vi "BPVI.vi"() -> ()   [LabVIEW 2014]
panel:
  in  "Array":void[](array[numeric])
  in  "Z-Expected":dbl
  in  "Y-Expected":dbl
  in  "X-Expected":dbl
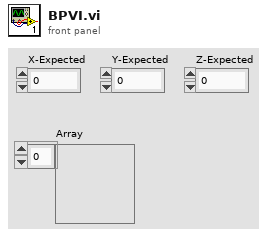
[diagram p1: front panel]
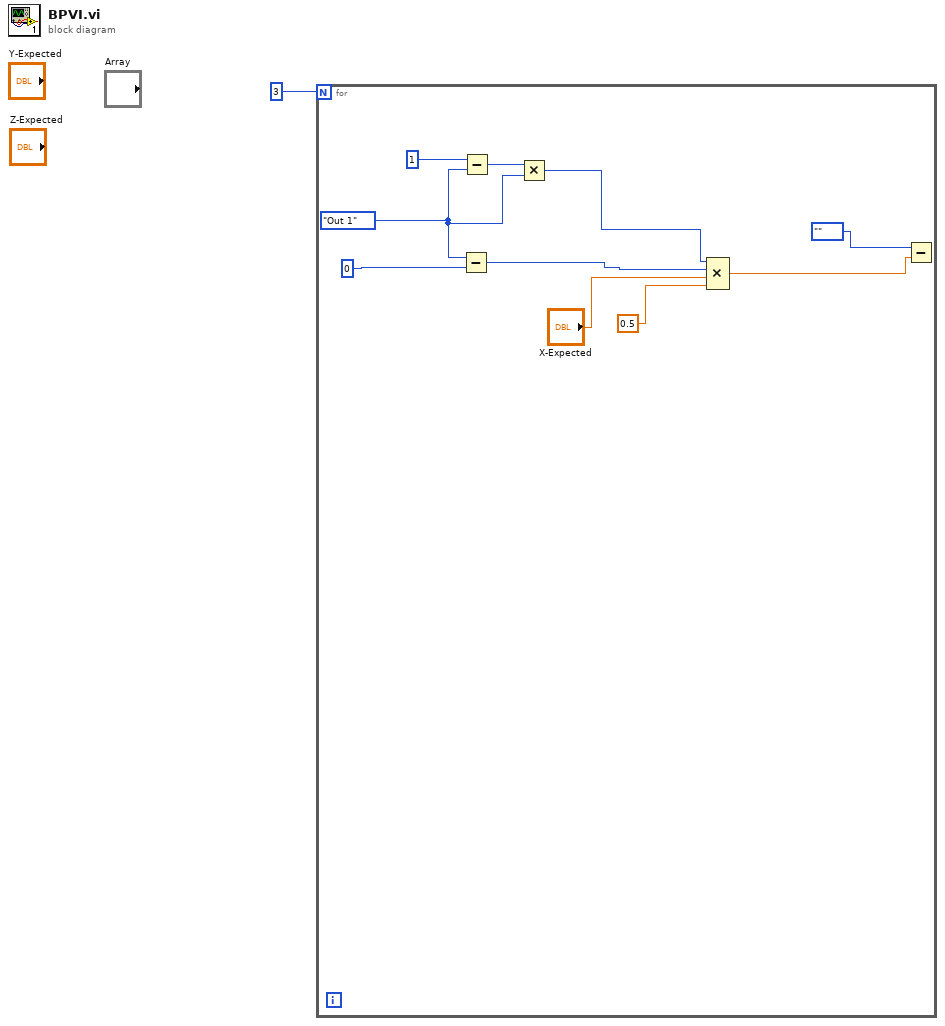
[diagram p0: block diagram]
diagram:
  n1 = for {
    N: 3 -> [_]
    w4 = enum16{"Out 1"}."Out 1"
    n2 = Subtract(x=w4, y=0) -> (x-y=w8:i32)
    n3 = Subtract(x=1, y=w4) -> (x-y=w3:i32)
    n4 = Multiply(x=w3, y=w4) -> (x*y=w7:i32)
    n5 = Compound Arithmetic op=MULTIPLY(w7, w8, "X-Expected", 0.5) -> (w11:dbl)
    n6 = Subtract(x=enum16{""}."", y=w11) -> ()  [unwired: 1 out]
  }
